vi "AB_API Deploy.vi"(8 "error in (no error)":errorcluster, 11 "Build in":refnum<class "AB_Build.lvclass">) -> (0 "error out":errorcluster, 3 "Build out":refnum<class "AB_Build.lvclass">)   [LabVIEW 2020]
uses:
  <vilib>/AppBuilder/AB_Classes/Build/AB_Build.lvclass
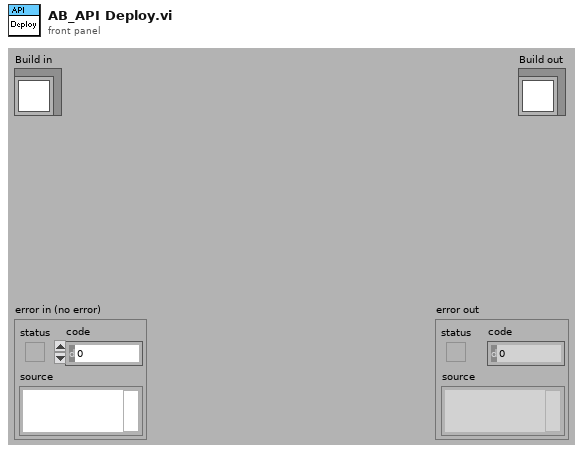
[diagram p1: front panel]
types:
  T1 = typedef "AB_Build.ctl" = cluster{"buildSpecName":string, "buildSpecDescription":string, "destinations":refnum<class "AB_Destination.lvclass">[], "exclusionOption":T2, "defaultLanguage":string, "supportedLanguages":string[], "excludedDirectories":path[], "buildContext":refnum<vi>, "buildObject":T3, "preview":bool, "programatic":bool, "progressBarEvents":T4, "userLog_Path":path, "preActionID":string, "preAction_Path":path, "postActionID":string, "postAction_Path":path, "eng_checkForBrokenVIs?":bool, "eng_verboseLinkerErrors?":bool, "localDest_Path":path, "targetDest_Path":path, "removeVIObject":u16, "cache":refnum<class "PreviewCache.lvclass">, "use cache":bool, "previewCache_ID":string, "buildCache_ID":string, "eng_TempLocalDest_Path":path, "eng_collectDependencies?":bool, "versionInfo":cluster{"buildVersion":cluster{"major":u16, "minor":u16, "patch":u16, "build":u16}, "autoIncrement":bool}, "eng_enableVIChecksums":bool}
  T2 = typedef "AB_Exclusion_Option.ctl" = cluster{"typedefs":bool, "polymorphicVIs":bool, "unusedLibraryItems":bool, "modifyLibraryFile":bool, "edit-timeDependencies":bool, "inlineVIs":bool, "dependent PPLs":bool, "dependent DLLs":bool}
  T3 = typedef "ItemRef.ctl" = u64
  T4 = typedef "provcom_ProgressBar_Events.ctl" = cluster{"newJob":refnum<user-event>, "newItem":refnum<user-event>, "errorMsg":T5, "cancel":refnum<user-event>}
  T5 = typedef "mxLvBuildError.ctl" = refnum<user-event>
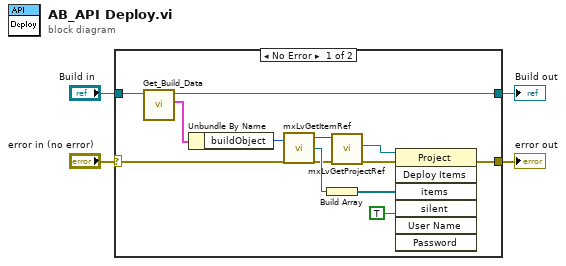
[diagram p0: block diagram]
diagram:
  n1 = case shown="No Error" "error in (no error)" {
    selector: "error in (no error)" -> [w5 w19]
    tunnel: "Build in" -> [w8 w18]
    tunnel: [w7 w18] -> w3
    tunnel: [w6 w19] -> w2
    frame No Error {
      n2 = call <vilib>:"Get_Build_Data.vi"("Class in"=w8) -> ("data"=w17:T1, "Class out"=w7:refnum<class "AB_Build.lvclass">)  [unwired: 8 in, 1 out]
      n3 = Unbundle By Name(w17) -> ("buildObject"=w16:T3)
      n4 = call <resource>:"mxLvGetItemRef.vi"("Item"=w16, "error in"=w5) -> ("Item"=w12:T3, "Item Refnum"=w15:refnum<vi>, "error out"=w11:errorcluster)
      n5 = Build Array(w15) -> (w14:refnum<vi>[])
      n6 = call <resource>:"mxLvGetProjectRef.vi"("error in"=w11, "Item"=w12) -> ("error out"=w9:errorcluster, "Project Refnum"=w10:refnum<vi>)  [unwired: 7 in, 1 out]
      n7 = invoke class="Project" method="Deploy Items"(reference=w10, error in=w9, "items"=w14, "silent"=TRUE ("Silent")) -> (error out=w6:errorcluster)  [unwired: 3 in, 6 out]
    }
    frame Error {
    }
  }
  "Build out" <- w3
  "error out" <- w2
